vi "myRIO_BRig_RT_comm_webdav_uploadReceived_check.vi"(11 "input_dataName":string="dataExp") -> (1 "output_Iexist":bool, 2 "output_dataPath":path)   [LabVIEW 2014]
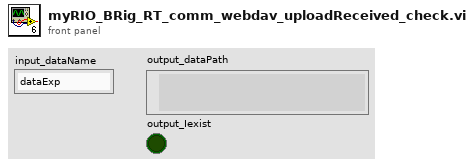
[diagram p1: front panel]
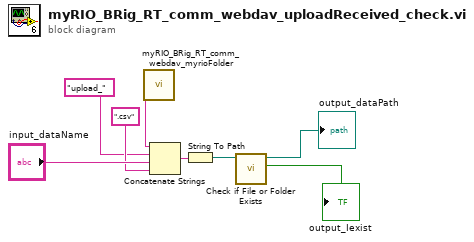
[diagram p0: block diagram]
diagram:
  n1 = call "myRIO_BRig_RT_comm_webdav_myrioFolder.vi"() -> ("output_myrioFolder"=w6:string)  [unwired: 11 in]
  n2 = Concatenate Strings(w6, "upload_" ("string"), "input_dataName", ".csv" ("string")) -> (w4:string)
  n3 = String To Path(string=w4) -> (path=w3:path)
  n4 = call <vilib>:"Check if File or Folder Exists.vi"("path"=w3) -> ("file or folder exists?"=→"output_Iexist":bool, "dup path"=→"output_dataPath":path)  [unwired: 8 in, 1 out]
